vi "macro_SwerveModStatePosNew4.vi"   [LabVIEW 2019, in "Trajectory_Library.lvlib"]
uses:
  Trajectory_Library.lvlib
types:
  T1 = typedef "Trajectory_Library.lvlib/ROTATION2D.ctl" = cluster{"VALUE":dbl, "COS":dbl, "SIN":dbl}
  T2 = typedef "Trajectory_Library.lvlib/SWERVE_DRIVE_MODULE_STATE.ctl" = cluster{"Speed":dbl, "Angle":T1}
  T3 = typedef "Trajectory_Library.lvlib/SWERVE_DRIVE_MODULE_POSITION.ctl" = cluster{"Distance":dbl, "Angle":T1, "P":bool}
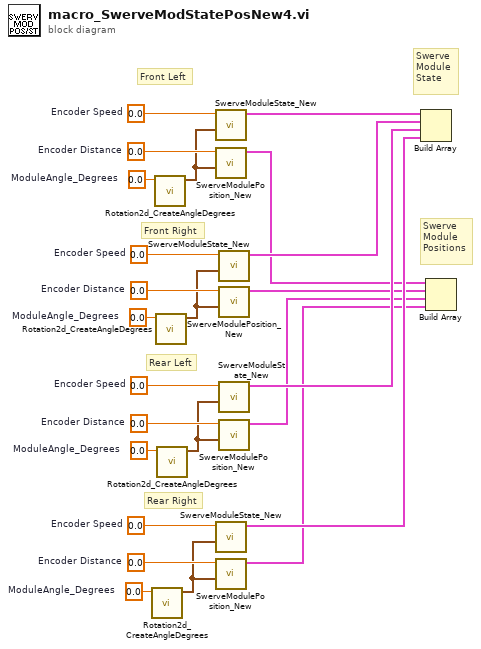
[diagram p0: block diagram]
diagram:
  w8 = 0.0  # Encoder Distance
  w9 = 0.0  # Encoder Distance
  w10 = 0.0  # Encoder Distance
  w12 = 0.0  # Encoder Distance
  w16 = 0.0  # ModuleAngle_Degrees
  w17 = 0.0  # Encoder Speed
  w18 = 0.0  # ModuleAngle_Degrees
  w19 = 0.0  # Encoder Speed
  w20 = 0.0  # ModuleAngle_Degrees
  w21 = 0.0  # Encoder Speed
  w23 = 0.0  # ModuleAngle_Degrees
  w24 = 0.0  # Encoder Speed
  # "Swerve\nModule\nPositions"
  # "Front Left"
  # "Swerve\nModule\nState"
  # "Rear Right"
  # "Rear Left"
  # "Front Right"
  n1 = call "Rotation2d_CreateAngleDegrees.vi"("Angle_Degrees"=w16) -> ("ROTATION"=w1:T1)  [unwired: 10 in]
  n2 = call "Rotation2d_CreateAngleDegrees.vi"("Angle_Degrees"=w23) -> ("ROTATION"=w4:T1)  [unwired: 10 in]
  n3 = call "Rotation2d_CreateAngleDegrees.vi"("Angle_Degrees"=w20) -> ("ROTATION"=w3:T1)  [unwired: 10 in]
  n4 = call "Rotation2d_CreateAngleDegrees.vi"("Angle_Degrees"=w18) -> ("ROTATION"=w2:T1)  [unwired: 10 in]
  n5 = call "SwerveModuleState_New.vi"("ROTATION"=w4, "Speed"=w24) -> ("SWERVE_DRIVE_MODULE_STATE"=w22:T2)  [unwired: 9 in]
  n6 = call "SwerveModulePosition_New.vi"("ROTATION"=w4, "Distance"=w12) -> ("SWERVE_DRIVE_MODULE_POSITION"=w11:T3)  [unwired: 9 in]
  n7 = call "SwerveModuleState_New.vi"("ROTATION"=w1, "Speed"=w17) -> ("SWERVE_DRIVE_MODULE_STATE"=w13:T2)  [unwired: 9 in]
  n8 = call "SwerveModulePosition_New.vi"("ROTATION"=w1, "Distance"=w8) -> ("SWERVE_DRIVE_MODULE_POSITION"=w5:T3)  [unwired: 9 in]
  n9 = call "SwerveModuleState_New.vi"("ROTATION"=w3, "Speed"=w21) -> ("SWERVE_DRIVE_MODULE_STATE"=w15:T2)  [unwired: 9 in]
  n10 = call "SwerveModulePosition_New.vi"("ROTATION"=w3, "Distance"=w10) -> ("SWERVE_DRIVE_MODULE_POSITION"=w7:T3)  [unwired: 9 in]
  n11 = call "SwerveModuleState_New.vi"("ROTATION"=w2, "Speed"=w19) -> ("SWERVE_DRIVE_MODULE_STATE"=w14:T2)  [unwired: 9 in]
  n12 = call "SwerveModulePosition_New.vi"("ROTATION"=w2, "Distance"=w9) -> ("SWERVE_DRIVE_MODULE_POSITION"=w6:T3)  [unwired: 9 in]
  n13 = Build Array(w22, w15, w14, w13) -> ()  [unwired: 1 out]
  n14 = Build Array(w11, w7, w6, w5) -> ()  [unwired: 1 out]
